vi "Read Math Result.vi"(8 "error in (no error)":errorcluster, 10 "Channel (0: Channel 1)":i32(ring) items=["Channel 1", "Channel 2"], 11 "VISA resource name":refnum<visa-resource-name>) -> (0 "error out":errorcluster, 2 "Math Result Data":T1, 3 "VISA resource name out":refnum<visa-resource-name>)   [LabVIEW 2020, in "Agilent B2900 Series.lvlib"]
doc: "Calculate specified math expression and return the result.\n\nNote:\nIf the math expression contains some measurement results, measurement may be performed many times to obtain the result. For example, measurement must be performed twice to get result of the following math expression.\nmath expression =(CURR[1]-CURR[0])"
uses:
  Agilent B2900 Series.lvlib
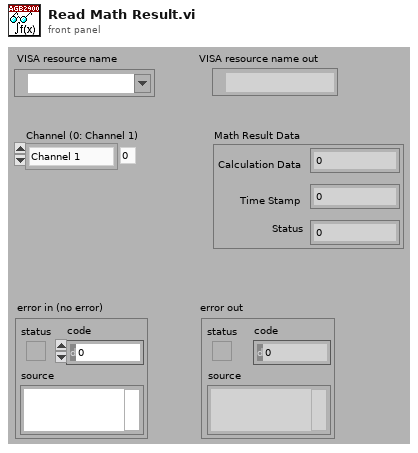
[diagram p1: front panel]
types:
  T1 = cluster{"Calculation Data":dbl, "Time Stamp":dbl, "Status":dbl}
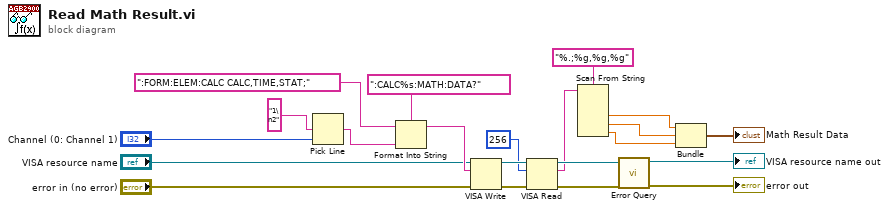
[diagram p0: block diagram]
diagram:
  n1 = Pick Line(multi-line string="1\n2" ("string (\"\")"), line index="Channel (0: Channel 1)") -> (output string=w8:string)  [unwired: 1 in]
  n2 = Format Into String(format string=":CALC%s:MATH:DATA?", initial string=":FORM:ELEM:CALC CALC,TIME,STAT;", w8) -> (resulting string=w21:string)  [unwired: 1 in, 1 out]
  n3 = VISA Write(VISA resource name="VISA resource name", write buffer=w21, error in (no error)="error in (no error)") -> (VISA resource name out=w15:refnum<visa-resource-name>, error out=w14:errorcluster)  [unwired: 1 out]
  n4 = VISA Read(VISA resource name=w15, byte count=u32 256, error in (no error)=w14) -> (VISA resource name out=w12:refnum<visa-resource-name>, read buffer=w2:string, error out=w13:errorcluster)  [unwired: 1 out]
  n5 = Scan From String(format string="%.;%g,%g,%g", input string=w2) -> (output 1=w3:dbl, output 2=w1:dbl, output 3=w5:dbl)  [unwired: 5 in, 3 out]
  n6 = call "Error Query.vi"("error in (no error)"=w13, "VISA resource name"=w12) -> ("error out"=→"error out":errorcluster, "VISA resource name out"=→"VISA resource name out":refnum<visa-resource-name>)  [unwired: 6 in, 2 out]
  n7 = Bundle(w3, w1, w5) -> (→"Math Result Data":cluster{dbl, dbl, dbl})  [unwired: 1 in]
